vi "OKN_CPG.vi"() -> ()   [LabVIEW 2016]
panel:
  out "EyeVelocities":cluster{dbl, "Eye position":dbl, dbl, dbl}(graph)
  out "Cereb 2":cluster{dbl, "PC Right":dbl, dbl}(graph)
  out "Cereb":cluster{dbl, "PC Right":dbl, dbl}(graph)
  in  "Log?":bool
  in  "Cere?":bool
  in  "Light?":bool
  in  "Period":bool=TRUE
  out "SimPars":T1
  in  "stop":bool
  out "Log File name":string="DataLog__27Feb15p55"
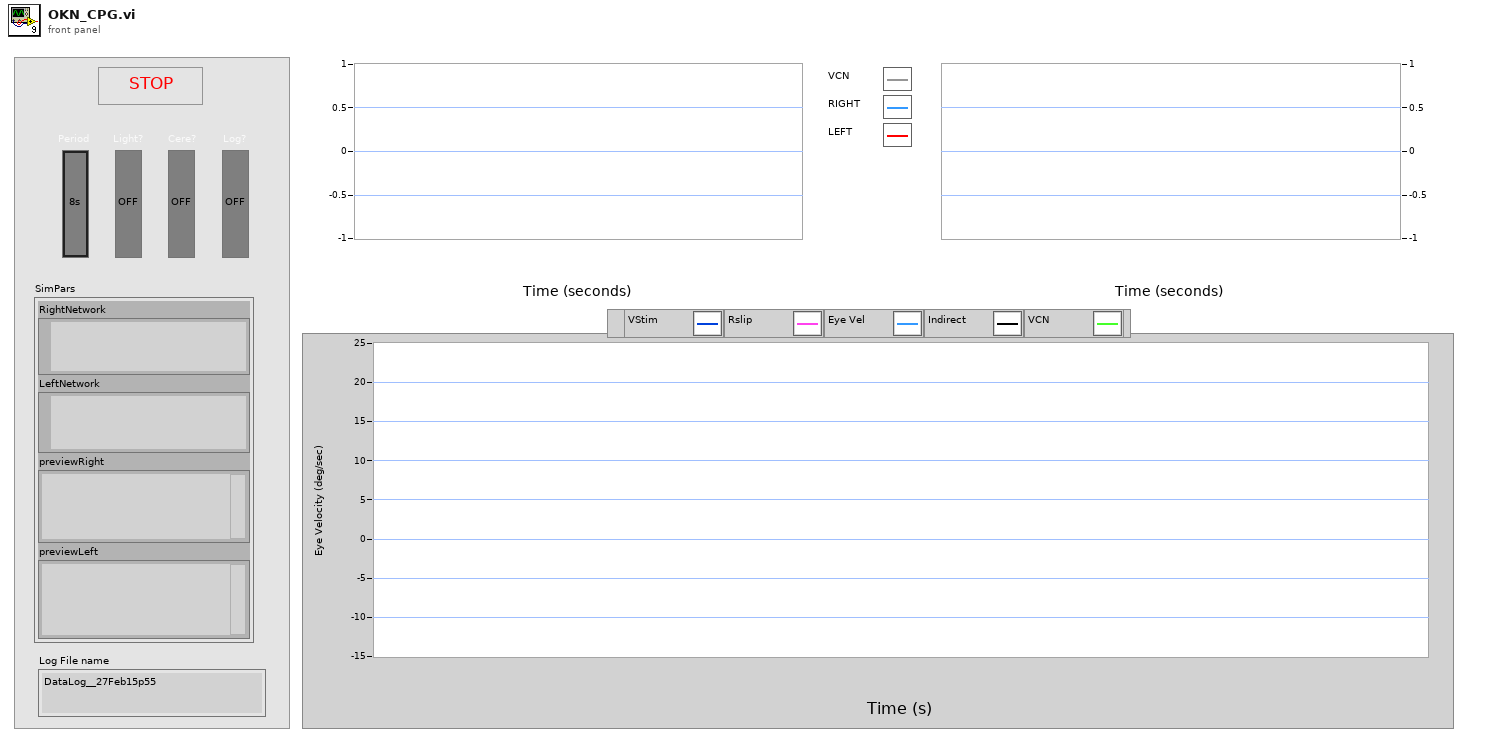
[diagram p1: front panel]
types:
  T1 = cluster{"RightNetwork":path, "LeftNetwork":path, "previewRight":string, "previewLeft":string}
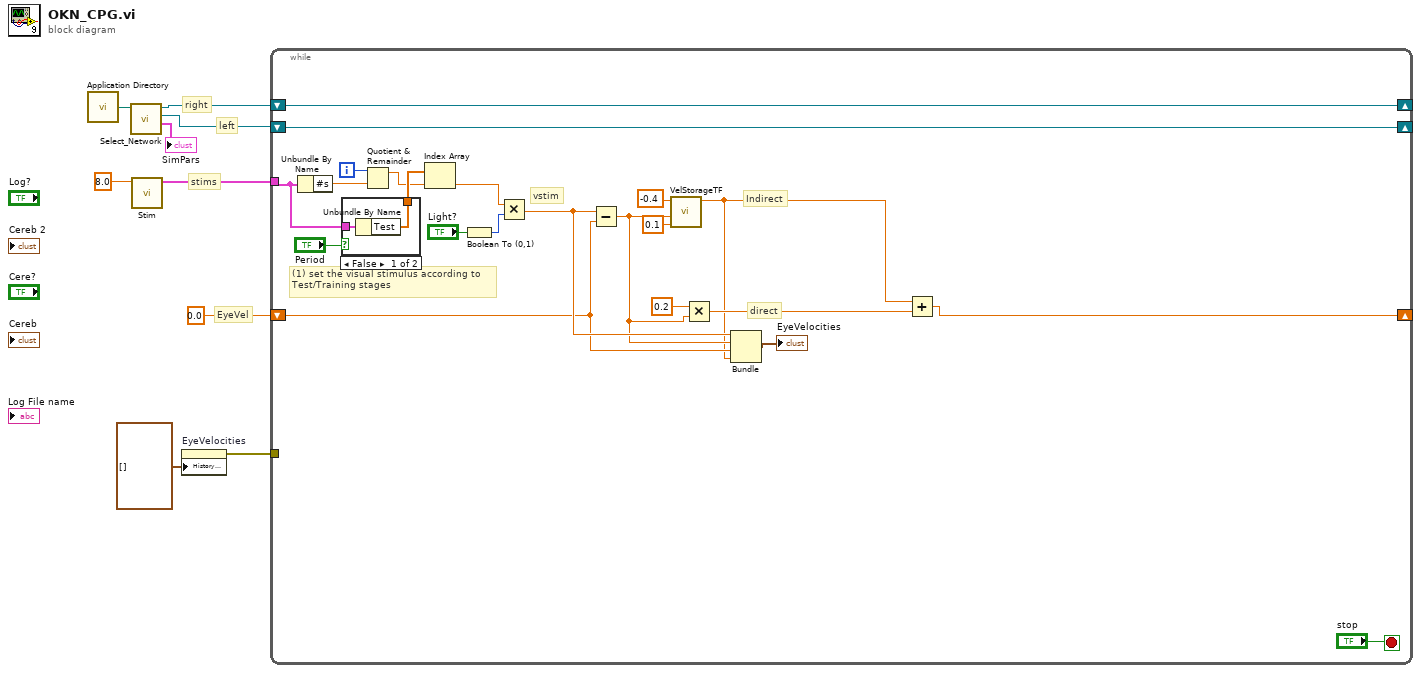
[diagram p0: block diagram]
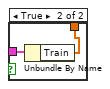
[diagram p2: hidden frame]
diagram:
  # "EyeVel"
  # "stims"
  # "left"
  # "right"
  n1 = call <vilib>:"Application Directory.vi"() -> ("Application Directory"=w9:path)
  n2 = call "Select_Network.vi"("base path"=w9) -> ("SimPars"=→"SimPars":T1, "CNN Left"=w6:refnum<class "CNN.lvclass">, "CNN Right"=w7:refnum<class "CNN.lvclass">)  [unwired: 7 in, 1 out]
  n3 = call "Stim.vi"("Tstim ON"=8.0) -> ("Vstim"=w4:cluster{"Test":dbl[], "Train":dbl[], "#s":dbl})  [unwired: 10 in]
  n4 = property on="EyeVelocities" class="WFChart (strict)"("History Data"=cluster{dbl, "Eye position":dbl, dbl, dbl}[] []) -> (error out=w2:errorcluster)  [unwired: 2 in, 1 out]
  n5 = while {
    shift-right: [w17] -> _
    shift-left: w7 -> [w17]
    shift-right: [w16] -> _
    shift-left: w6 -> [w16]
    tunnel: w4 -> [w27]
    shift-right: [w19] -> _
    shift-left: 0.0 -> [w12]
    tunnel: w2 -> [_]
    i -> [w29]
    stop <- "stop" stop-if-true
    # "direct"
    # "Indirect"
    # "(1) set the visual stimulus according to\nTest/Training stages"
    # "vstim"
    n6 = Unbundle By Name(w27) -> ("#s"=w30:dbl)
    n7 = case shown="False" "Period" {
      tunnel: w27 -> [w33 w35]
      tunnel: [w32 w34] -> w26
      frame False {
        n8 = Unbundle By Name(w33) -> ("Test"=w32:dbl[])
      }
      frame True {
        n9 = Unbundle By Name(w35) -> ("Train"=w34:dbl[])
      }
    }
    n10 = Quotient & Remainder(x=w29, y=w30) -> (x-y*floor(x/y)=w15:dbl)  [unwired: 1 out]
    n11 = Index Array(array=w26, index=w15) -> (element=w23:dbl)
    n12 = Boolean To (0,1)(Boolean="Light?") -> (0, 1=w24:i16)
    n13 = Multiply(x=w23, y=w24) -> (x*y=w14:dbl)
    n14 = Subtract(x=w14, y=w12) -> (x-y=w13:dbl)
    n15 = call "VelStorageTF.vi"("Int. Step (ms)"=0.1, "Retinal Slip"=w13, "Leak cnt"=-0.4) -> ("Eye position"=w11:dbl)  [unwired: 8 in]
    n16 = Multiply(x=0.2, y=w13) -> (x*y=w18:dbl)
    n17 = Bundle(w14, w13, w12, "Eye position"=w11) -> (→"EyeVelocities":cluster{dbl, dbl, dbl, "Eye position":dbl})  [unwired: 1 in]
    n18 = Add(x=w11, y=w18) -> (x+y=w19:dbl)
  }
